vi "subVI_example.vi"(9 "amplitude":dbl, 10 "frequency":dbl, 11 "Ring":u16) -> (3 "signal out":waveform(dbl))   [LabVIEW 2026]
uses:
  <vilib>/measure/NI_MABase.lvlib
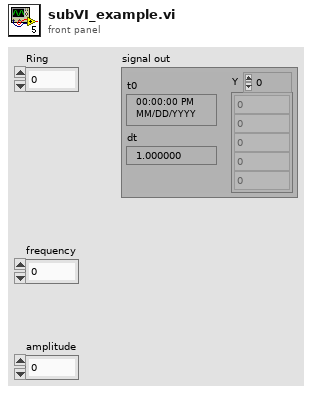
[diagram p1: front panel]
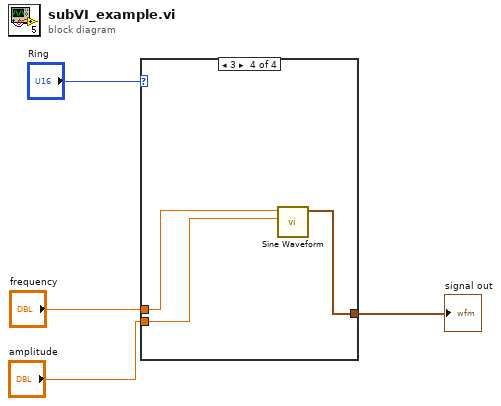
[diagram p0: block diagram]
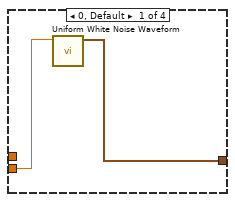
[diagram p2: hidden frame]
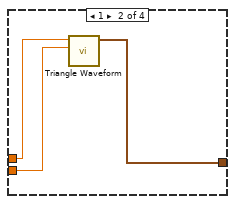
[diagram p3: hidden frame]
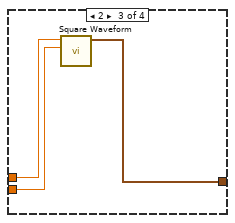
[diagram p4: hidden frame]
diagram:
  n1 = case shown="3" "Ring" {
    tunnel: "frequency" -> [_ w9 w12 w15]
    tunnel: "amplitude" -> [w5 w8 w11 w14]
    tunnel: [w6 w7 w10 w13] -> w4
    frame 0, Default {
      n2 = call <vilib>:"Uniform White Noise Waveform.vi"("amplitude"=w5) -> ("signal out"=w6:waveform(dbl))  [unwired: 9 in, 1 out]
    }
    frame 1 {
      n3 = call <vilib>:"Triangle Waveform.vi"("amplitude"=w8, "frequency"=w9) -> ("signal out"=w7:waveform(dbl))  [unwired: 8 in, 1 out]
    }
    frame 2 {
      n4 = call <vilib>:"Square Waveform.vi"("amplitude"=w11, "frequency"=w12) -> ("signal out"=w10:waveform(dbl))  [unwired: 8 in, 1 out]
    }
    frame 3 {
      n5 = call <vilib>:"Sine Waveform.vi"("amplitude"=w14, "frequency"=w15) -> ("signal out"=w13:waveform(dbl))  [unwired: 8 in, 1 out]
    }
  }
  "signal out" <- w4
